vi "AutoFileCreatorMain.vi"() -> ()   [LabVIEW 2017]
uses:
  Utils/FilePath.vi
  <vilib>/Utility/inputDevices.llb/mouseAcquire.vi
  <vilib>/xml/NI_XML.lvlib
  <resource>/objmgr/DOMUserDefRef.rc
panel:
  in  "LocalFileNames":string[](array[string])=["1A.txt", "1B.txt", "1C.txt", "1D.txt", "2A.txt", "2B.txt", "2C.txt", "2D.txt", "3A.txt", "3B.txt", "3C.txt", "3D.txt", "4A.txt", "4B.txt", "4C.txt", "4D.txt"]
  out "standard output":string
  out "standard error":string="NI Linux Real-Time (run mode)\n\nLog in with your NI-Auth credentials.\n\n"
  in  "LocalFiles":i32(listbox)=2
  in  "SaveToLocal":bool
  in  "LoadFromLocal":bool
  in  "ExportToRobot":bool
  out "XML With IDs":string="<Sequential ID=\"1\">\n</Sequential>"
  in  "Commands":i32(listbox)=-1
  out "XML":string="<Sequential>\n</Sequential>"
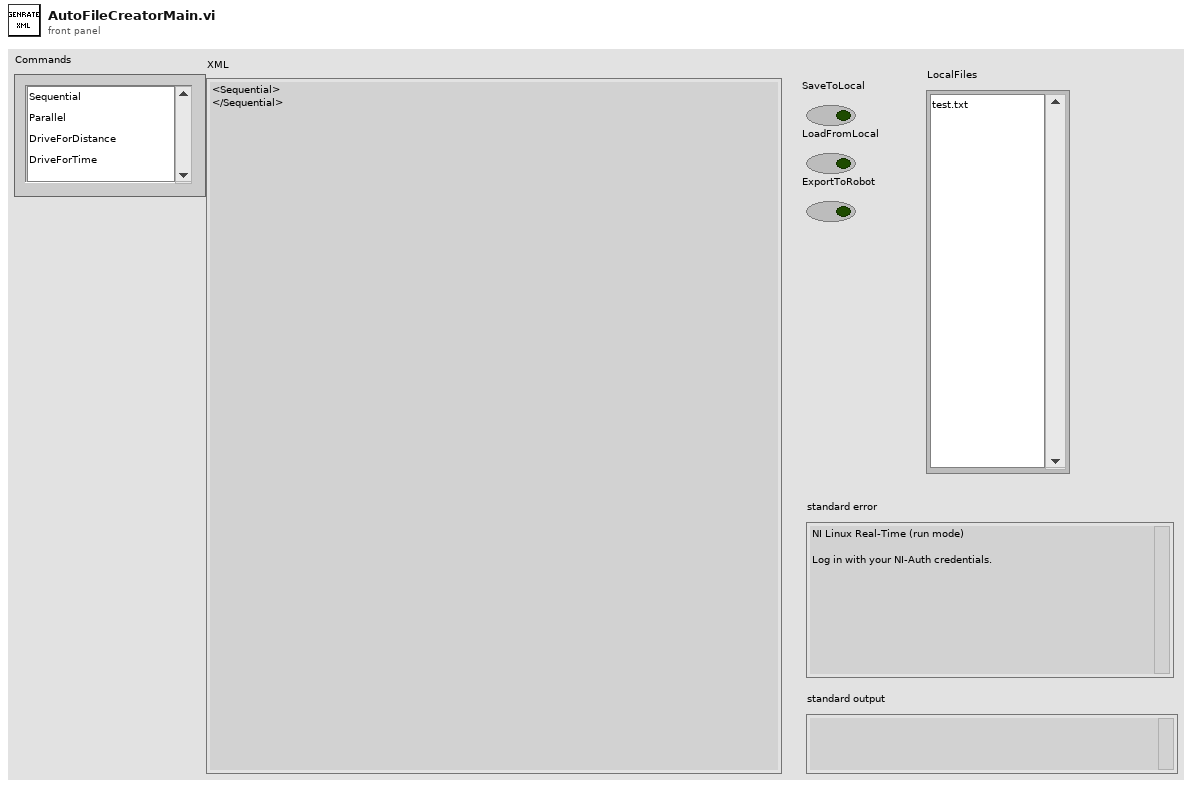
[diagram p1: front panel]
types:
  T1 = cluster{"Horizontal":i32, "Vertical":i32, "Scrolling":i32}
  T2 = typedef "eventvkey.ctl" = enum16{"ASCII", "Enter", "Return", "Shift", "Ctrl", "Alt", "Cmd", "Opt", "Caps", "NumLock", "Clear", "Break", "Up", "Down", "Left", "Right", "Insert", "Delete", "Home", "End", "PageUp", "PageDown", "Escape", "Help", "Pause", "ScrollLock", "F1", "F2", "F3", "F4", "F5", "F6", "F7", "F8", "F9", "F10", "F11", "F12", "F13", "F14", "F15", "F16", "F17", "F18", "F19", "F20", "F21", "F22", "F23", "F24", "Play", "VolumeUp", "VolumeDown", "Mute", "Two Byte Char"}
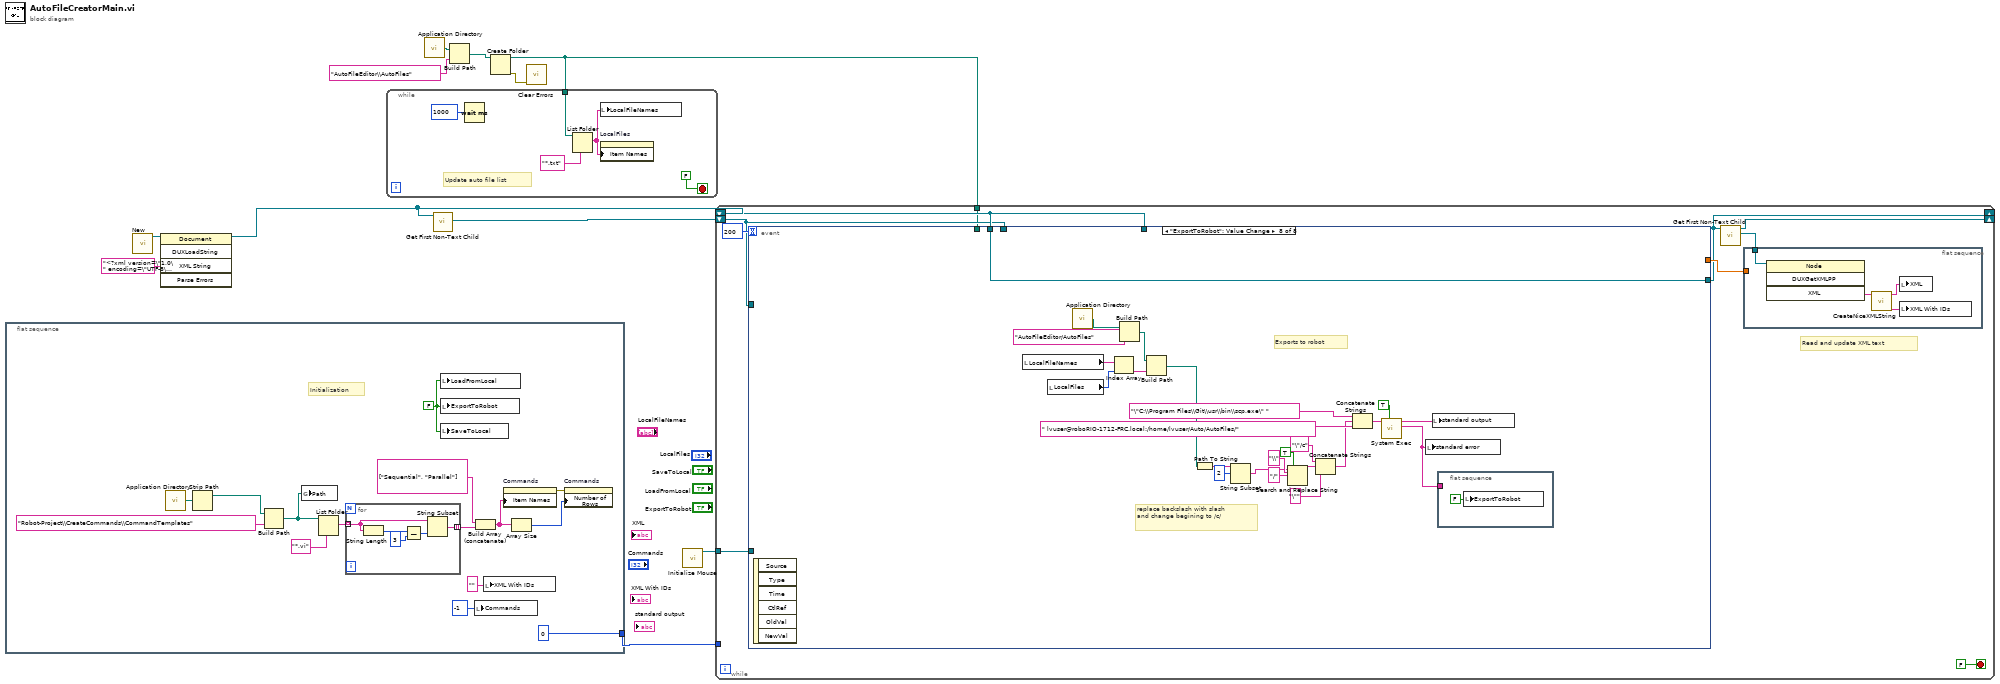
[diagram p0: block diagram]
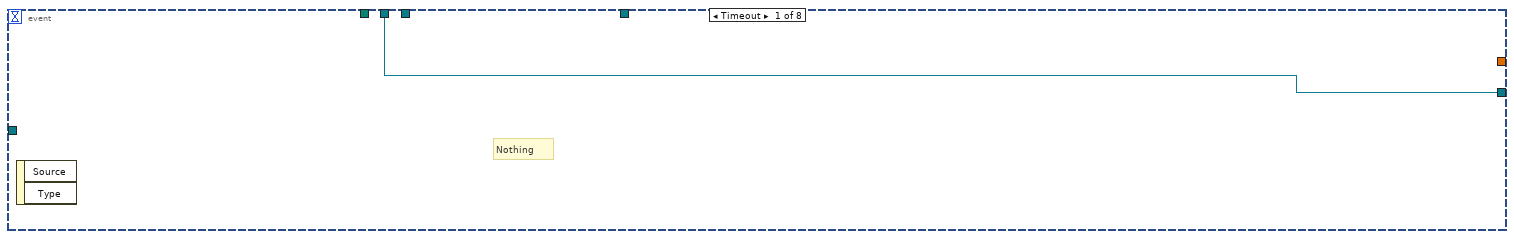
[diagram p2: hidden frame]
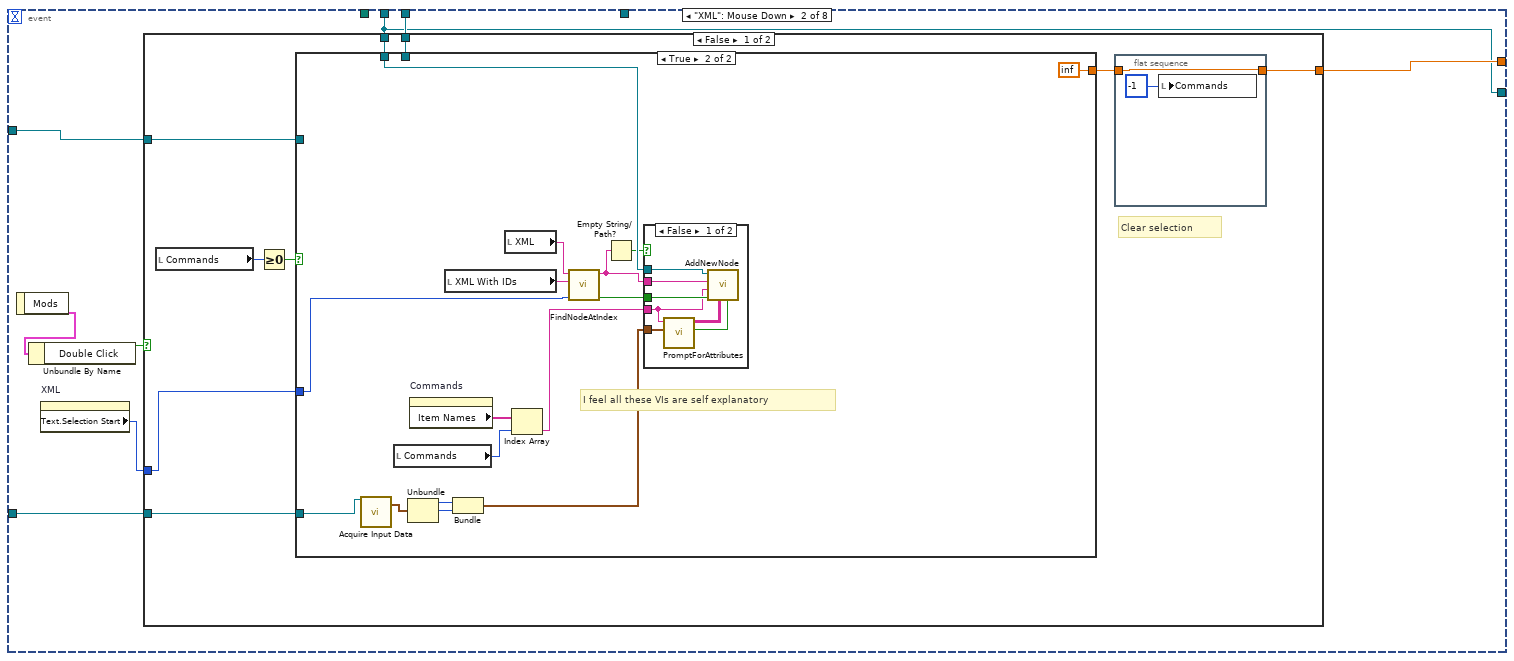
[diagram p3: hidden frame]
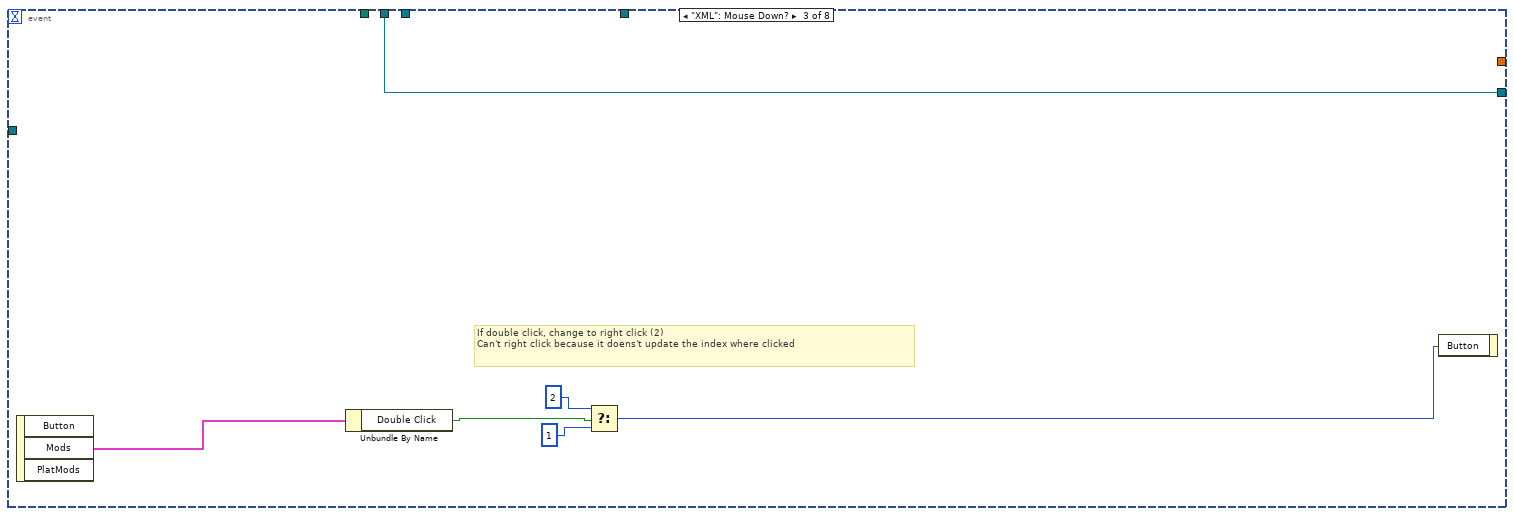
[diagram p7: hidden frame]
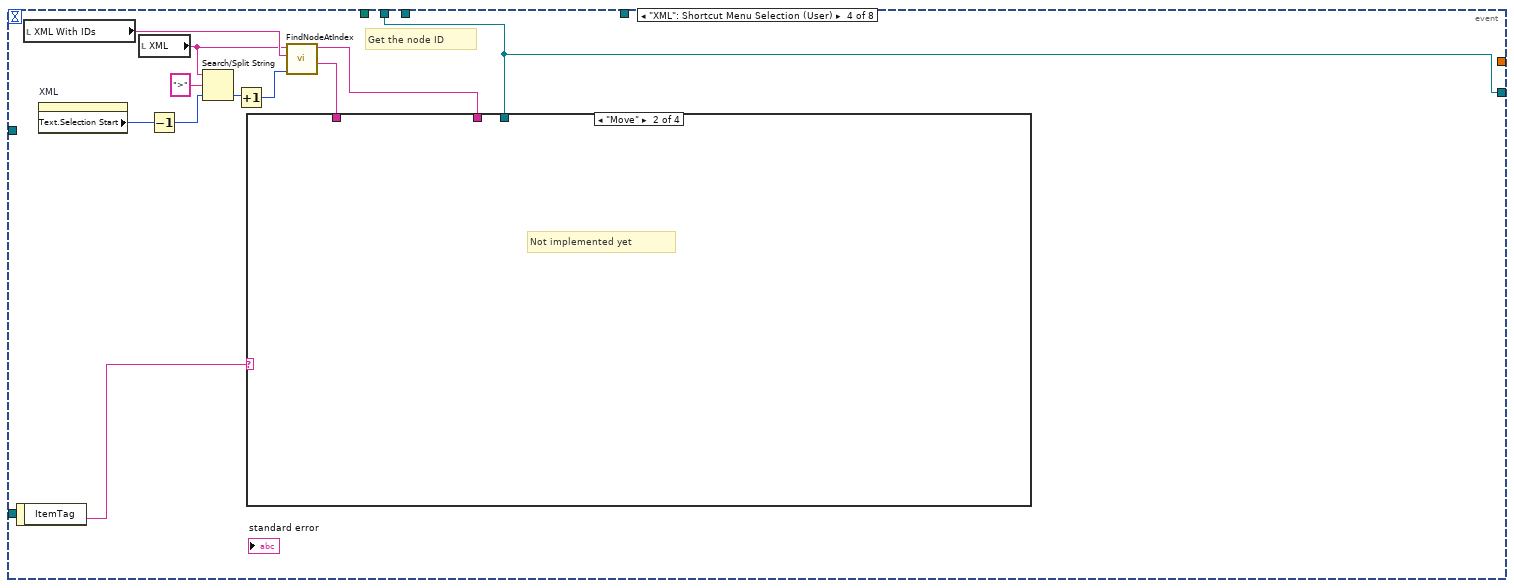
[diagram p8: hidden frame]
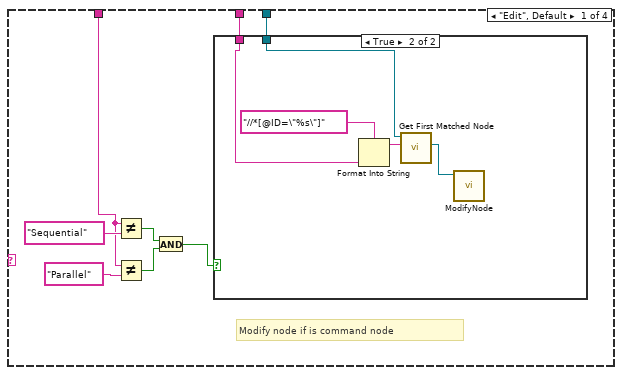
[diagram p9: hidden frame]
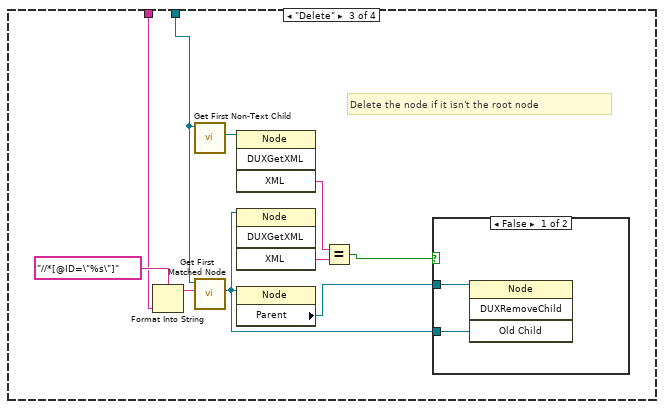
[diagram p11: hidden frame]
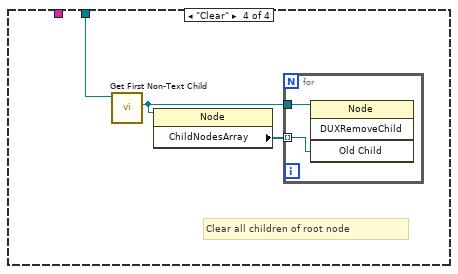
[diagram p13: hidden frame]
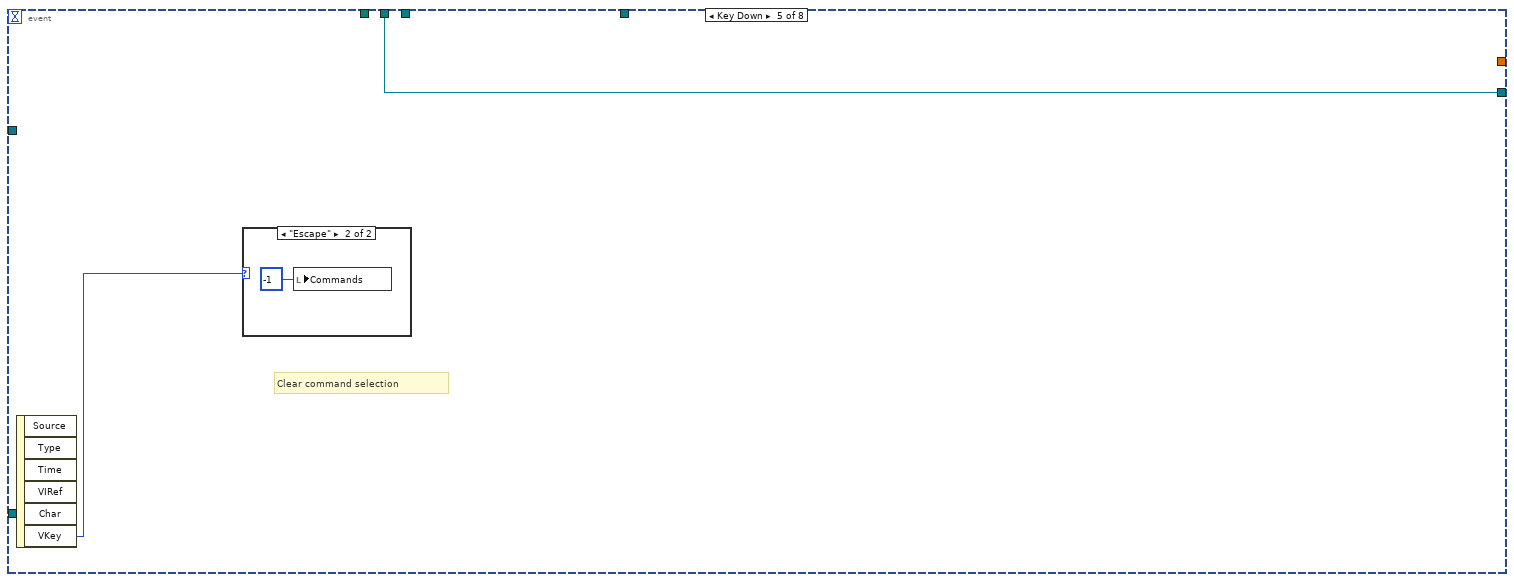
[diagram p14: hidden frame]
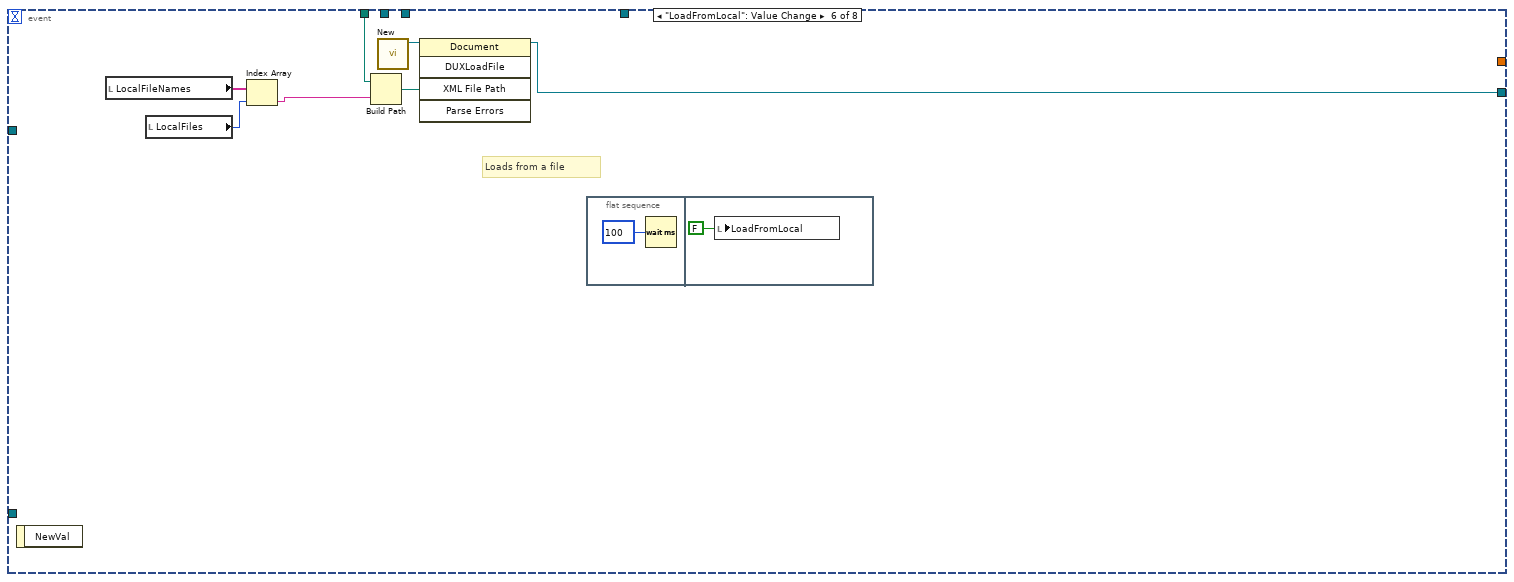
[diagram p16: hidden frame]
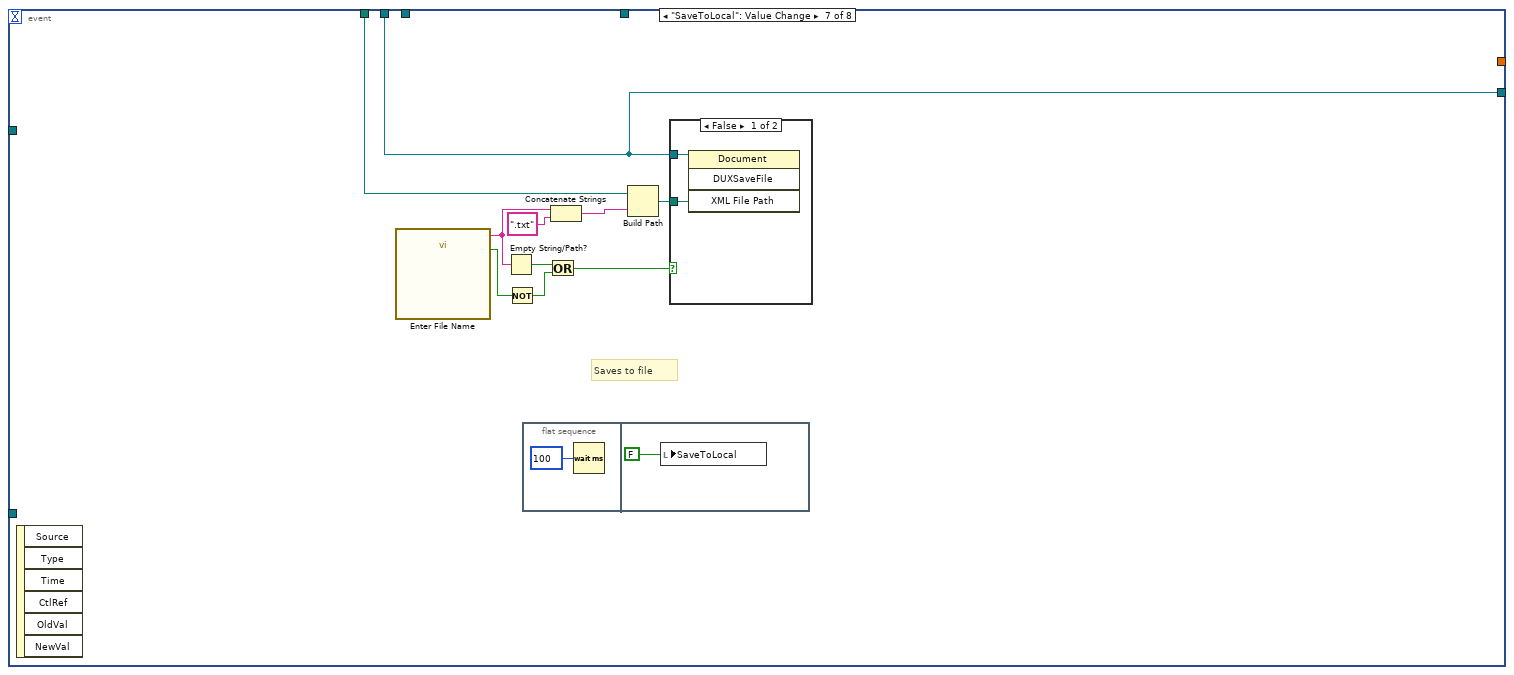
[diagram p17: hidden frame]
diagram:
  n1 = flat-sequence {
    tunnel: [0] -> w11
    frame #0 {
      w15 = FALSE ("SaveToLocal")
      # "Initialization"
      n2 = call <vilib>:"Application Directory.vi"() -> ("Application Directory"=w12:path)
      n3 = Strip Path(path=w12) -> (stripped path=w14:path)  [unwired: 1 out]
      n4 = Build Path(base path=w14, name or relative path="Robot-Project\\CreateCommands\\CommandTemplates") -> (appended path=w13:path)
      n5 = global write "FilePath.vi" "Path"(w13) -> ()
      n6 = List Folder(path=w13, pattern="*.vi") -> (filenames=w19:string[])  [unwired: 2 in, 3 out]
      n7 = for {
        tunnel: w19 -> [w31] mode=indexing
        tunnel: [w27] -> w20 mode=indexing
        n8 = String Length(string=w31) -> (length=w30:i32)
        n9 = Subtract(x=w30, y=3) -> (x-y=w28:i32)
        n10 = String Subset(string=w31, length (rest)=w28) -> (substring=w27:string)  [unwired: 1 in]
      }
      n11 = local write "LoadFromLocal"(w15) -> ()
      n12 = local write "ExportToRobot"(w15) -> ()
      n13 = local write "SaveToLocal"(w15) -> ()
      n14 = local write "Commands"(-1 ("Active Row:Active Row Number")) -> ()
      n15 = Build Array (concatenate)(string[] ["Sequential", "Parallel"], w20) -> (w21:string[])
      n16 = local write "XML With IDs"("" ("XML With IDs")) -> ()
      n17 = property on="Commands" class="LstBox (strict)"("Item Names"=w21) -> (error out=w23:errorcluster)  [unwired: 2 in, 1 out]
      n18 = Array Size(array=w21) -> (size(s)=w22:i32)
      n19 = property on="Commands" class="LstBox (strict)"(error in=w23, "Number of Rows"=w22) -> ()  [unwired: 1 in, 2 out]
    }
  }
  n20 = call <vilib>:"New.vi"() -> ("DOM document out"=w10:refnum<k20>)  [unwired: 8 in, 1 out]
  n21 = invoke class="Document" method="DUXLoadString"(reference=w10, "XML String"="<?xml version=\"1.0\" encoding=\"UTF-8\"?><Sequential ID=\"1\"></Sequential>") -> (reference out=w9:refnum<k20>)  [unwired: 3 in, 4 out]
  n22 = call <vilib>:"Application Directory.vi"() -> ("Application Directory"=w4:path)
  n23 = call <vilib>:"Get First Non-Text Child.vi"("node in"=w9) -> ("child node"=w8:refnum<k20>)  [unwired: 7 in, 3 out]
  n24 = Build Path(base path=w4, name or relative path="AutoFileEditor\\AutoFiles") -> (appended path=w1:path)
  n25 = Create Folder(path (use dialog)=w1) -> (created path=w3:path, error out=w2:errorcluster)  [unwired: 2 in, 1 out]
  n26 = while {
    tunnel: w3 -> [w32]
    stop <- FALSE stop-if-true
    # "Update auto file list"
    n27 = Wait (ms)(milliseconds to wait=u32 1000) -> ()  [unwired: 1 out]
    n28 = List Folder(path=w32, pattern="*.txt") -> (filenames=w33:string[])  [unwired: 2 in, 3 out]
    n29 = local write "LocalFileNames"(w33) -> ()
    n30 = property on="LocalFiles" class="LstBox (strict)"("Item Names"=w33) -> ()  [unwired: 2 in, 2 out]
  }
  n31 = call <vilib>:"Clear Errors.vi"("error in (no error)"=w2) -> ()  [unwired: 5 in, 2 out]
  n32 = call <vilib>:"Initialize Mouse.vi"() -> ("device ID"=w7:refnum<k1>)  [unwired: 10 in, 1 out]
  n33 = while {
    tunnel: w11 -> [_]
    shift-right: [w38] -> _
    shift-left: w9 -> [w42]
    shift-right: [w40] -> _
    shift-left: w8 -> [w41]
    tunnel: w7 -> [w43]
    tunnel: w3 -> [w37]
    stop <- FALSE stop-if-true
    # "Read and update XML text"
    n34 = event shown="[7] \"ExportToRobot\": Value Change" {
      selector: _ -> [_ _ _ _ _ _ _ _]
      dyn-events: _ -> [_ _ _ _ _ _ _ _]
      timeout: 200 -> [_ _ _ _ _ _ _ _]
      tunnel: w41 -> [_ w59 _ _ _ _ _ _]
      tunnel: w42 -> [w51 w52 w94 w100 w141 _ w154 w168]
      tunnel: w41 -> [_ w58 _ _ _ _ _ _]
      tunnel: [_ w57 _ _ _ _ _ _] -> w44
      tunnel: w43 -> [_ w56 _ _ _ _ _ _]
      tunnel: w42 -> [_ _ _ _ _ _ _ _]
      tunnel: [w51 w52 w94 w100 w141 w146 w154 w168] -> w38
      tunnel: w37 -> [_ _ _ _ _ w144 w153 _]
      event Timeout {
        # "Nothing"
        n35 = event-data() -> ()  [unwired: 1 in, 2 out]
      }
      event "XML": Mouse Down {
        n36 = event-data() -> ("Mods"=w55:cluster{"Double Click":bool, "Menu Key":bool})  [unwired: 1 in]
        n37 = Unbundle By Name(w55) -> ("Double Click"=w54:bool)
        n38 = property on="XML" class="Str"() -> ("Text.Selection Start"=w53:u32)  [unwired: 2 in, 2 out]
        n39 = case shown="False" w54 {
          tunnel: w59 -> [w66 _]
          tunnel: w52 -> [w65 _]
          tunnel: w58 -> [w64 _]
          tunnel: [w62 _] -> w57
          tunnel: w56 -> [w61 _]
          tunnel: w53 -> [w60 _]
          frame False {
            # "Clear selection"
            n40 = local read "Commands"() -> (w68:i32)
            n41 = Greater Or Equal To 0?(x=w68) -> (x >= 0?=w67:bool)
            n42 = case shown="True" w67 {
              tunnel: w66 -> [_ _]
              tunnel: w65 -> [_ w77]
              tunnel: w64 -> [_ _]
              tunnel: w60 -> [_ w81]
              tunnel: [_ inf] -> w63
              tunnel: w61 -> [_ w75]
              frame False {
              }
              frame True {
                # "I feel all these VIs are self explanatory"
                n43 = call-poly <vilib>:"Acquire Input Data.vi"("device ID"=w75) -> ("axis info"=w74:T1)  [unwired: 15 in, 3 out]
                n44 = local read "Commands"() -> (w83:i32)
                n45 = Unbundle(w74) -> ("Horizontal"=w73:i32, "Vertical"=w72:i32)  [unwired: 1 out]
                n46 = property on="Commands" class="LstBox (strict)"() -> ("Item Names"=w84:string[])  [unwired: 2 in, 2 out]
                n47 = local read "XML With IDs"() -> (w80:string)
                n48 = Bundle("Horizontal"=w73, "Vertical"=w72) -> (w69:cluster{"Horizontal":i32, "Vertical":i32})  [unwired: 1 in]
                n49 = local read "XML"() -> (w79:string)
                n50 = Index Array(array=w84, index=w83) -> (element=w76:string)
                n51 = call "FindNodeAtIndex.vi"("ClickIndex"=w81, "XML with IDs"=w80, "XML In"=w79) -> ("Insert as child not sibling"=w78:bool, "Node ID"=w71:string)  [unwired: 6 in, 1 out]
                n52 = Empty String/Path?(string/path=w71) -> (empty?=w70:bool)
                n53 = case shown="False" w70 {
                  tunnel: w78 -> [w91 _]
                  tunnel: w77 -> [w90 _]
                  tunnel: w76 -> [w87 _]
                  tunnel: w71 -> [w89 _]
                  tunnel: w69 -> [w88 _]
                  frame False {
                    n54 = call "PromptForAttributes.vi"("Mouse Coords"=w88, "New Node Name"=w87) -> ("Canceled"=w86:bool, "Attributes"=w85:string[][])  [unwired: 8 in]
                    n55 = call "AddNewNode.vi"("Cancel"=w86, "Attributes"=w85, "Insert As Child"=w91, "New Node Name"=w87, "Node ID"=w89, "DOM document"=w90) -> ()  [unwired: 6 in]
                  }
                  frame True {
                  }
                }
              }
            }
            n56 = flat-sequence {
              tunnel: w63 -> [w92]
              tunnel: [w92] -> w62
              frame #0 {
                n57 = local write "Commands"(-1 ("Active Row:Active Row Number")) -> ()
              }
            }
          }
          frame True {
            # "Leave double clicking to that other event case"
          }
        }
      }
      event "XML": Mouse Down? {
        # "If double click, change to right click (2)\nCan't right click because it doens't update the index where clicked"
        n58 = event-data() -> ("Mods"=w99:cluster{"Double Click":bool, "Menu Key":bool})  [unwired: 1 in, 2 out]
        n59 = Unbundle By Name(w99) -> ("Double Click"=w98:bool)
        n60 = Select(t=u16 2 ("Button"), s=w98, f=u16 1 ("Button")) -> (s? t:f=w95:u16)
        n61 = event-data("Button"=w95) -> ()  [unwired: 1 in, 1 out]
      }
      event "XML": Shortcut Menu Selection (User) {
        # "Get the node ID"
        n62 = event-data() -> ("ItemTag"=w105:string)  [unwired: 1 in]
        n63 = local read "XML With IDs"() -> (w102:string)
        n64 = property on="XML" class="Str"() -> ("Text.Selection Start"=w110:u32)  [unwired: 2 in, 2 out]
        n65 = local read "XML"() -> (w101:string)
        n66 = Decrement(x=w110) -> (x-1=w108:u32)
        n67 = Search/Split String(string=w101, search string/char (-)=">", offset (0)=w108) -> (offset of match=w106:i32)  [unwired: 2 out]
        n68 = Increment(x=w106) -> (x+1=w107:i32)
        n69 = call "FindNodeAtIndex.vi"("ClickIndex"=w107, "XML with IDs"=w102, "XML In"=w101) -> ("Node Name"=w103:string, "Node ID"=w104:string)  [unwired: 6 in, 1 out]
        n70 = case shown="\"Move\"" w105 {
          tunnel: w104 -> [w118 _ w131 _]
          tunnel: w100 -> [w117 _ w124 w138]
          tunnel: w103 -> [w114 _ _ _]
          frame "Edit", Default {
            # "Modify node if is command node"
            n71 = Not Equal?(x=w114, y="Sequential") -> (x != y?=w115:bool)
            n72 = Not Equal?(x=w114, y="Parallel") -> (x != y?=w112:bool)
            n73 = And(x=w115, y=w112) -> (x .and. y?=w111:bool)
            n74 = case shown="True" w111 {
              tunnel: w118 -> [_ w121]
              tunnel: w117 -> [_ w119]
              frame False {
              }
              frame True {
                n75 = Format Into String(format string="//*[@ID=\"%s\"]", w121) -> (resulting string=w123:string)  [unwired: 2 in, 1 out]
                n76 = call <vilib>:"Get First Matched Node.vi"("XPath expression"=w123, "node in"=w119) -> ("node result"=w120:refnum<k20>)  [unwired: 7 in, 2 out]
                n77 = call "ModifyNode.vi"("Node"=w120) -> ()  [unwired: 11 in]
              }
            }
          }
          frame "Move" {
            # "Not implemented yet"
          }
          frame "Delete" {
            # "Delete the node if it isn't the root node"
            n78 = Format Into String(format string="//*[@ID=\"%s\"]", w131) -> (resulting string=w133:string)  [unwired: 2 in, 1 out]
            n79 = call <vilib>:"Get First Non-Text Child.vi"("node in"=w124) -> ("child node"=w129:refnum<k20>)  [unwired: 7 in, 3 out]
            n80 = call <vilib>:"Get First Matched Node.vi"("XPath expression"=w133, "node in"=w124) -> ("node result"=w127:refnum<k20>)  [unwired: 7 in, 2 out]
            n81 = invoke class="Node" method="DUXGetXML"(reference=w129) -> ("XML"=w128:string)  [unwired: 3 in, 3 out]
            n82 = invoke class="Node" method="DUXGetXML"(reference=w127) -> ("XML"=w126:string)  [unwired: 3 in, 3 out]
            n83 = property class="Node"(reference=w127) -> ("Parent"=w130:refnum<k20>)  [unwired: 1 in, 2 out]
            n84 = Equal?(x=w128, y=w126) -> (x = y?=w125:bool)
            n85 = case shown="False" w125 {
              tunnel: w130 -> [w135 _]
              tunnel: w127 -> [w134 _]
              frame False {
                n86 = invoke class="Node" method="DUXRemoveChild"(reference=w135, "Old Child"=w134) -> ()  [unwired: 2 in, 4 out]
              }
              frame True {
              }
            }
          }
          frame "Clear" {
            # "Clear all children of root node"
            n87 = call <vilib>:"Get First Non-Text Child.vi"("node in"=w138) -> ("child node"=w136:refnum<k20>)  [unwired: 7 in, 3 out]
            n88 = property class="Node"(reference=w136) -> ("ChildNodesArray"=w137:refnum<k20>[])  [unwired: 1 in, 2 out]
            n89 = for {
              tunnel: w136 -> [w140]
              tunnel: w137 -> [w139] mode=indexing
              n90 = invoke class="Node" method="DUXRemoveChild"(reference=w140, "Old Child"=w139) -> ()  [unwired: 2 in, 4 out]
            }
          }
        }
      }
      event Key Down {
        # "Clear command selection"
        n91 = event-data() -> ("VKey"=w142:T2)  [unwired: 1 in, 5 out]
        n92 = case shown="\"Escape\"" w142 {
          frame "ASCII", Default {
          }
          frame "Escape" {
            n93 = local write "Commands"(-1 ("Active Row:Active Row Number")) -> ()
          }
        }
      }
      event "LoadFromLocal": Value Change {
        # "Loads from a file"
        n94 = event-data() -> ()  [unwired: 1 in, 1 out]
        n95 = local read "LocalFileNames"() -> (w150:string[])
        n96 = local read "LocalFiles"() -> (w149:i32)
        n97 = Index Array(array=w150, index=w149) -> (element=w145:string)
        n98 = Build Path(base path=w144, name or relative path=w145) -> (appended path=w148:path)
        n99 = call <vilib>:"New.vi"() -> ("DOM document out"=w147:refnum<k20>)  [unwired: 8 in, 1 out]
        n100 = invoke class="Document" method="DUXLoadFile"(reference=w147, "XML File Path"=w148) -> (reference out=w146:refnum<k20>)  [unwired: 3 in, 4 out]
        n101 = flat-sequence {
          frame #0 {
            n102 = Wait (ms)(milliseconds to wait=u32 100) -> ()  [unwired: 1 out]
          }
          frame #1 {
            n103 = local write "LoadFromLocal"(FALSE ("SaveToLocal")) -> ()
          }
        }
      }
      event "SaveToLocal": Value Change {
        # "Saves to file"
        n104 = event-data() -> ()  [unwired: 1 in, 6 out]
        n105 = call "Enter File Name"() -> ("File Name"=w156:string, "Enter"=w160:bool)  [unwired: 17 in, 1 out]
        n106 = Empty String/Path?(string/path=w156) -> (empty?=w162:bool)
        n107 = Not(x=w160) -> (.not. x?=w161:bool)
        n108 = flat-sequence {
          frame #0 {
            n109 = Wait (ms)(milliseconds to wait=u32 100) -> ()  [unwired: 1 out]
          }
          frame #1 {
            n110 = local write "SaveToLocal"(FALSE ("SaveToLocal")) -> ()
          }
        }
        n111 = Or(x=w162, y=w161) -> (x .or. y?=w155:bool)
        n112 = Concatenate Strings(w156, ".txt" ("string")) -> (w158:string)
        n113 = Build Path(base path=w153, name or relative path=w158) -> (appended path=w157:path)
        n114 = case shown="False" w155 {
          tunnel: w154 -> [w164 _]
          tunnel: w157 -> [w163 _]
          frame False {
            n115 = invoke class="Document" method="DUXSaveFile"(reference=w164, "XML File Path"=w163) -> ()  [unwired: 2 in, 4 out]
          }
          frame True {
          }
        }
      }
      event "ExportToRobot": Value Change {
        # "Exports to robot"
        # "replace backslash with slash\nand change begining to /c/"
        n116 = event-data() -> ()  [unwired: 1 in, 6 out]
        n117 = local read "LocalFileNames"() -> (w188:string[])
        n118 = local read "LocalFiles"() -> (w187:i32)
        n119 = call <vilib>:"Application Directory.vi"() -> ("Application Directory"=w167:path)
        n120 = Index Array(array=w188, index=w187) -> (element=w189:string)
        n121 = Build Path(base path=w167, name or relative path="AutoFileEditor/AutoFiles") -> (appended path=w190:path)
        n122 = Build Path(base path=w190, name or relative path=w189) -> (appended path=w171:path)
        n123 = Path To String(path=w171) -> (string=w178:string)
        n124 = String Subset(string=w178, offset (0)=2) -> (substring=w176:string)  [unwired: 1 in]
        n125 = Search and Replace String(replace all?=TRUE ("replace all? (F)"), input string=w176, search string="\\", replace string="/" ("replace string (\"\")")) -> (result string=w175:string)  [unwired: 4 in, 3 out]
        n126 = Concatenate Strings("\"/c" ("string"), w175, "\"" ("string")) -> (w173:string)
        n127 = Concatenate Strings("\"C:\\Program Files\\Git\\usr\\bin\\scp.exe\" " ("command line"), w173, " lvuser@roboRIO-1712-FRC.local:/home/lvuser/Auto/AutoFiles/" ("string")) -> (w182:string)
        n128 = call <vilib>:"System Exec.vi"("wait until completion? (T)"=TRUE, "command line"=w182) -> ("standard error"=w169:string, "standard output"=w170:string)  [unwired: 6 in, 2 out]
        n129 = local write "standard error"(w169) -> ()
        n130 = local write "standard output"(w170) -> ()
        n131 = flat-sequence {
          tunnel: w169 -> [_]
          frame #0 {
            n132 = local write "ExportToRobot"(FALSE ("ExportToRobot")) -> ()
          }
        }
      }
    }
    n133 = call <vilib>:"Get First Non-Text Child.vi"("node in"=w38) -> ("child node"=w39:refnum<k20>, "node out"=w40:refnum<k20>)  [unwired: 7 in, 2 out]
    n134 = flat-sequence {
      tunnel: w44 -> [_]
      tunnel: w39 -> [w47]
      frame #0 {
        n135 = invoke class="Node" method="DUXGetXMLPP"(reference=w47) -> ("XML"=w48:string)  [unwired: 3 in, 3 out]
        n136 = call "CreateNiceXMLString.vi"("XML In"=w48) -> ("XML String With IDs"=w49:string, "XML String Human Readable"=w50:string)  [unwired: 9 in]
        n137 = local write "XML"(w50) -> ()
        n138 = local write "XML With IDs"(w49) -> ()
      }
    }
  }
